vi "Color-Senser-Dtermine-Pro_Api.vi"(8 "Error In":errorcluster, 11 "HiTechnicColorSensorV2 Ref In":cluster{"I2C Ref Out":T2}) -> (0 "Error Out":errorcluster, 1 "Green or Saturation":i32, 2 "對應顏色":enum16{"黃", "紅", "綠", "藍", "黑", "無"}(ring), 3 "HiTechnicColorSensorV2 Ref Out":cluster{"I2C Ref Out":T2}, 4 "Red or Hue":i32, 5 "當前顏色值":T1(array[cluster]))   [LabVIEW 2019]
uses:
  Variable/Indentify-Consequent.vi
  <vilib>/myRIO/Common/Instrument Driver Framework/myRIO v1.0/DIO/typedefs/DIO Channels Enum.ctl
  <vilib>/myRIO/Common/Instrument Driver Framework/myRIO v1.0/DIO/typedefs/DIO Channels List.ctl
  <vilib>/myRIO/Common/Instrument Driver Framework/Utilities/typedefs/Generic FPGA Reference.ctl
  <vilib>/myRIO/Common/Instrument Driver Framework/Utilities/typedefs/myRIO v1.0 Reference.ctl
  <vilib>/myRIO/Common/Instrument Driver Framework/Utilities/typedefs/Hardware Version Enum.ctl
  <vilib>/myRIO/Common/Instrument Driver Framework/Utilities/typedefs/myRIO Generic Hardware Reference.ctl
  <vilib>/myRIO/Instrument Drivers/Onboard IO/DIO/typedefs/DIO Reference.ctl
  <vilib>/myRIO/Instrument Drivers/Onboard IO/DIO/DIO.lvlib
  <vilib>/myRIO/Instrument Drivers/Onboard IO/DIO/vis/Write.vi
  <vilib>/userDefined/High Color/nirio_resource_hc.ctl
  <vilib>/myRIO/Common/Instrument Driver Framework/myRIO v1.0/DIO/vis/myRIO v1.1 Open DIO.vi
  <vilib>/myRIO/Instrument Drivers/Onboard IO/DIO/vis/myRIO DIO Open.xnode
  <vilib>/myRIO/Common/Instrument Driver Framework/Utilities/vis/Is FPGA Ref Available.vi
  <vilib>/myRIO/Express VI/Onboard Devices/LED/LED Express VI.xnode
  <vilib>/myRIO/Common/Instrument Driver Framework/myRIO v1.0/I2C/typedefs/I2C Channels Enum.ctl
  <vilib>/myRIO/Instrument Drivers/Onboard IO/I2C/typedefs/I2C Transfer Rate.ctl
  <vilib>/myRIO/Instrument Drivers/Onboard IO/I2C/I2C.lvlib
  <vilib>/myRIO/Instrument Drivers/Onboard IO/I2C/typedefs/I2C Configuration.ctl
  <vilib>/myRIO/Instrument Drivers/Onboard IO/I2C/typedefs/I2C Reference.ctl
panel:
  in  "Stop":bool
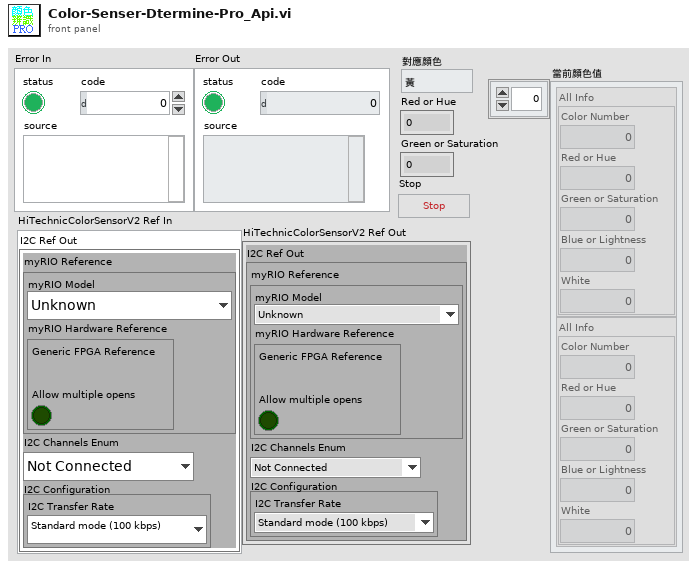
[diagram p1: front panel]
types:
  T1 = cluster{"All Info":cluster{"Color Number":i32, "Red or Hue":i32, "Green or Saturation":i32, "Blue or Lightness":i32, "White":i32}}[]
  T2 = typedef "I2C.lvlib/I2C Reference.ctl" = cluster{"myRIO Reference":T3, "I2C Channels Enum":T7, "I2C Configuration":T8}
  T3 = typedef "myRIO Generic Hardware Reference.ctl" = cluster{"myRIO Model":T4, "myRIO Hardware Reference":T5}
  T4 = typedef "Hardware Version Enum.ctl" = enum16{"Unknown", "myRIO-1900", "myRIO-1950", "roboRIO", "NI ELVIS RIO CM", "ELVIS III"}
  T5 = typedef "myRIO v1.0 Reference.ctl" = cluster{"Generic FPGA Reference":T6, "Allow multiple opens":bool}
  T6 = typedef "Generic FPGA Reference.ctl" = refnum<k20>
  T7 = typedef "I2C Channels Enum.ctl" = enum16{"Not Connected", "A/I2C", "B/I2C", "I2C/I2C"}
  T8 = typedef "I2C.lvlib/I2C Configuration.ctl" = cluster{"I2C Transfer Rate":T9}
  T9 = typedef "I2C.lvlib/I2C Transfer Rate.ctl" = enum16{"Standard mode (100 kbps)", "Fast mode (400 kbps)"}
  T10 = cluster{"All Info":cluster{"Color Number":i32, "Red or Hue":i32, "Green or Saturation":i32, "Blue or Lightness":i32, "White":i32}}
  T11 = typedef "DIO.lvlib/DIO Reference.ctl" = cluster{"myRIO Reference":T3, "DIO Channels List":T12}
  T12 = typedef "DIO Channels List.ctl" = T13[]
  T13 = typedef "DIO Channels Enum.ctl" = enum16{"Not Connected", "C/DIO0", "C/DIO1", "C/DIO2", "C/DIO3", "C/DIO4", "C/DIO5", "C/DIO6", "C/DIO7", "A/DIO0", "A/DIO1", "A/DIO2", "A/DIO3", "A/DIO4", "A/DIO5", "A/DIO6", "A/DIO7", "A/DIO8", "A/DIO9", "A/DIO10", "A/DIO11", "A/DIO12", "A/DIO13", "A/DIO14", "A/DIO15", "A/DIO16", "A/DIO17", "A/DIO18", "A/DIO19", "B/DIO0", "B/DIO1", "B/DIO2", "B/DIO3", "B/DIO4", "B/DIO5", "B/DIO6", "B/DIO7", "B/DIO8", "B/DIO9", "B/DIO10", "B/DIO11", "B/DIO12", "B/DIO13", "B/DIO14", "B/DIO15", "B/DIO16", "B/DIO17", "B/DIO18", "B/DIO19", "LED0", "LED1", "LED2", "LED3", "Button0", "DIO/DIO0", "DIO/DIO1", "DIO/DIO2", "DIO/DIO3", "DIO/DIO4", "DIO/DIO5", "DIO/DIO6", "DIO/DIO7", "DIO/DIO8", "DIO/DIO9", "SPI/CS0", "SPI/CS1", "SPI/CS2", "SPI/CS3", "LED RADIO (Green)", "LED RADIO (Red)", "LED COMM (Green)", "LED COMM (Red)", "LED MODE (Green)", "LED MODE (Red)"}
  T14 = typedef "nirio_resource_hc.ctl" = tag
  T15 = cluster{"Color Number":i32, "Red or Hue":i32, "Green or Saturation":i32, "Blue or Lightness":i32, "White":i32}
  T16 = cluster{"Color Number":dbl, "Red or Hue":dbl, "Green or Saturation":dbl, "Blue or Lightness":dbl, "White":dbl}
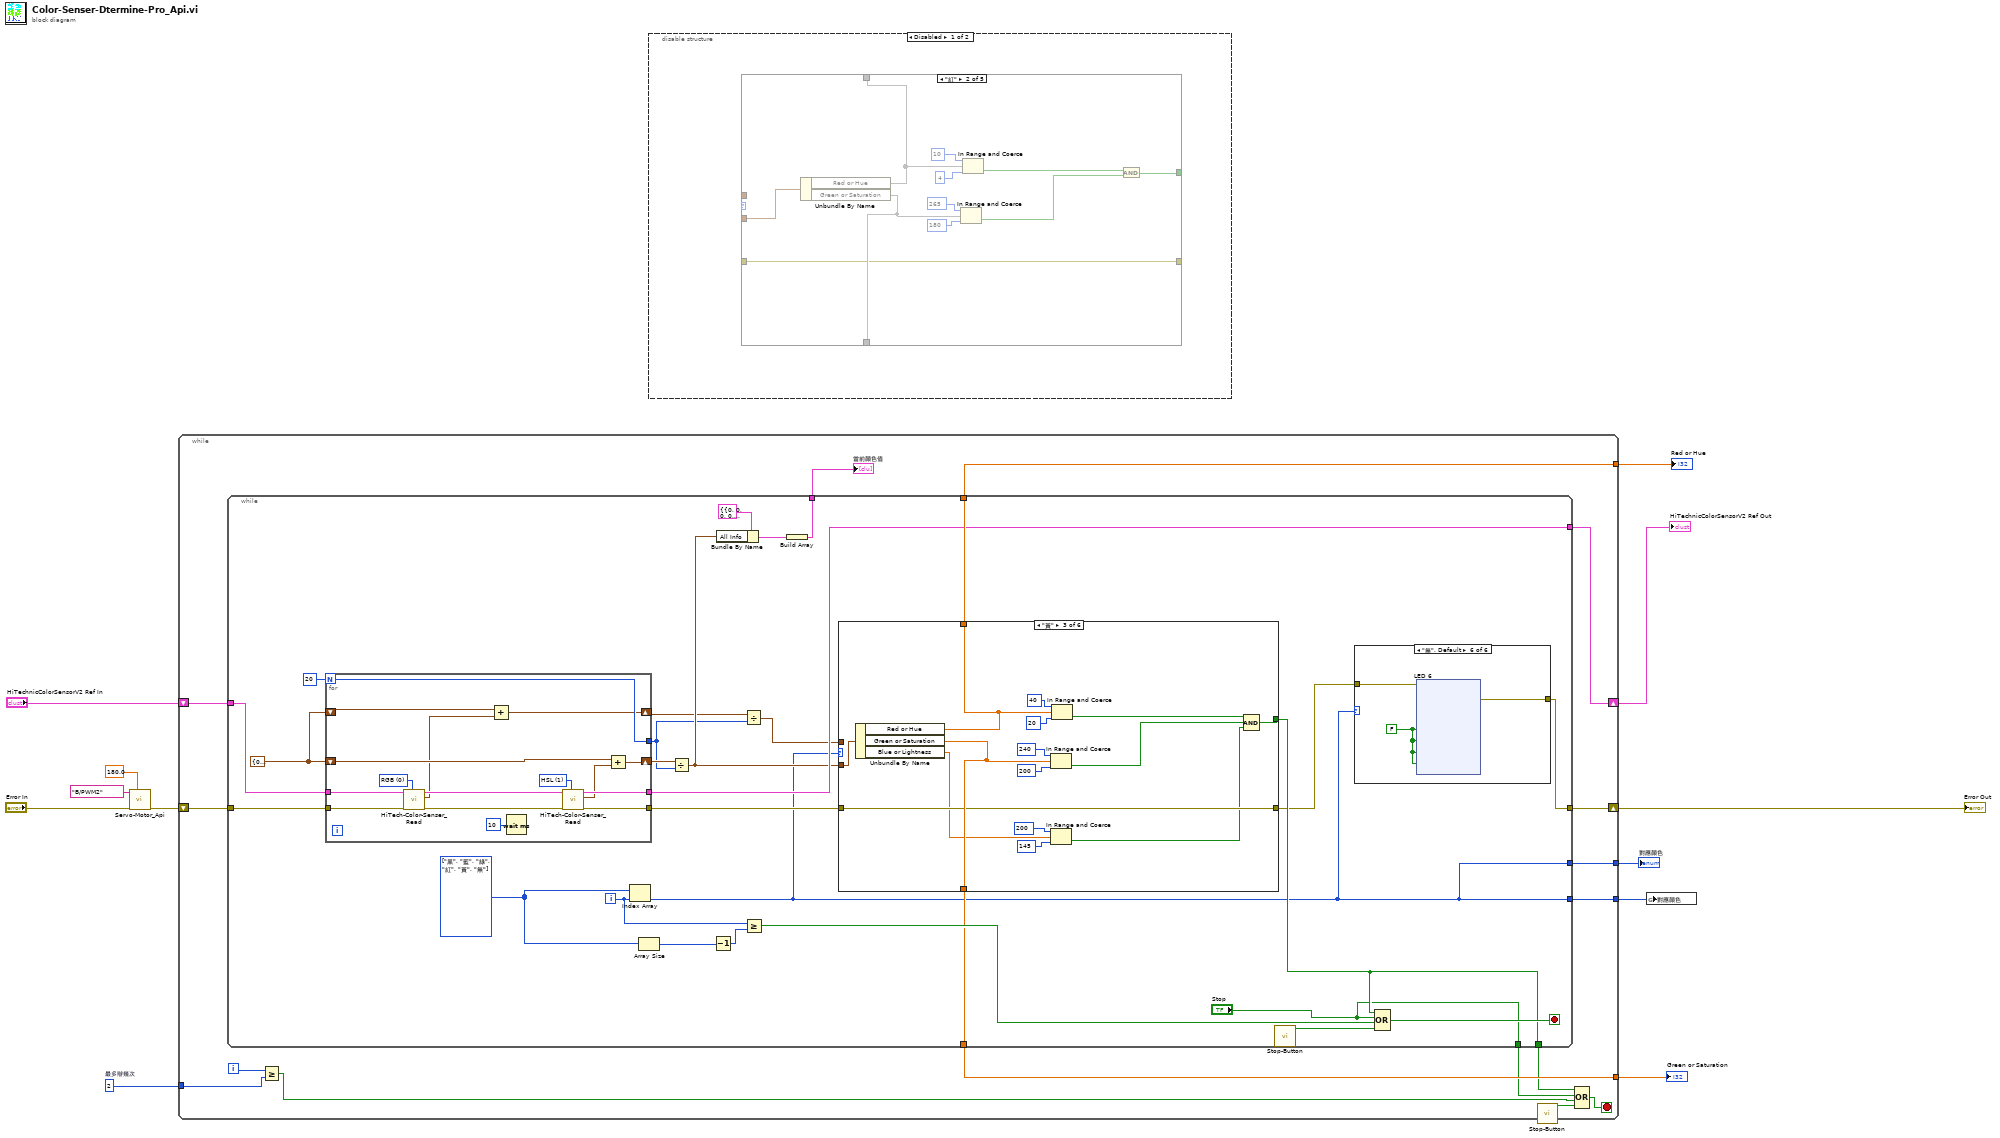
[diagram p0: block diagram]
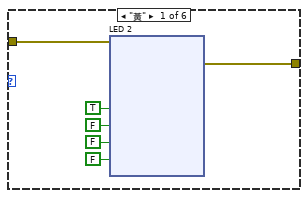
[diagram p2: hidden frame]
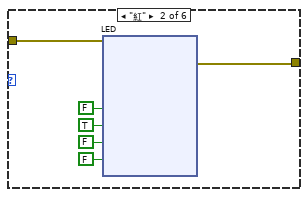
[diagram p3: hidden frame]
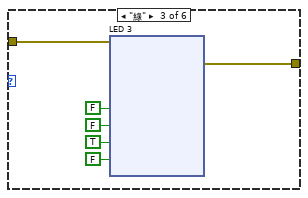
[diagram p4: hidden frame]
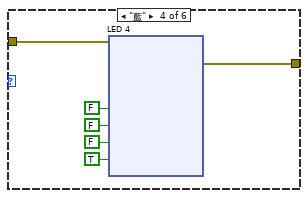
[diagram p5: hidden frame]
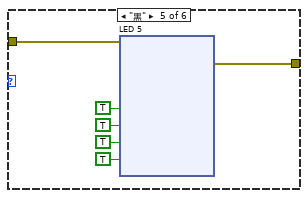
[diagram p6: hidden frame]
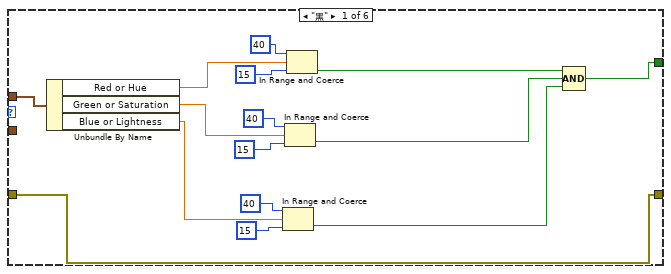
[diagram p7: hidden frame]
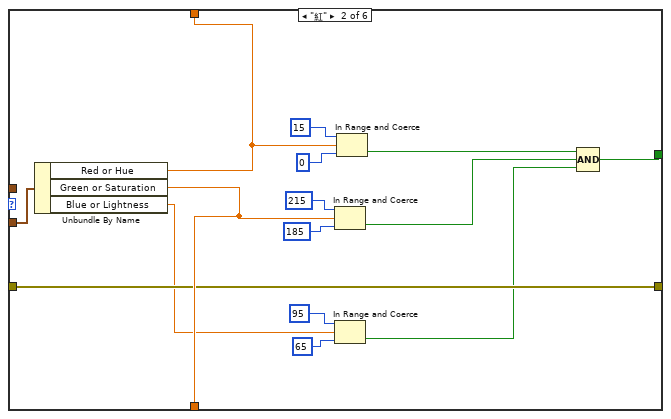
[diagram p8: hidden frame]
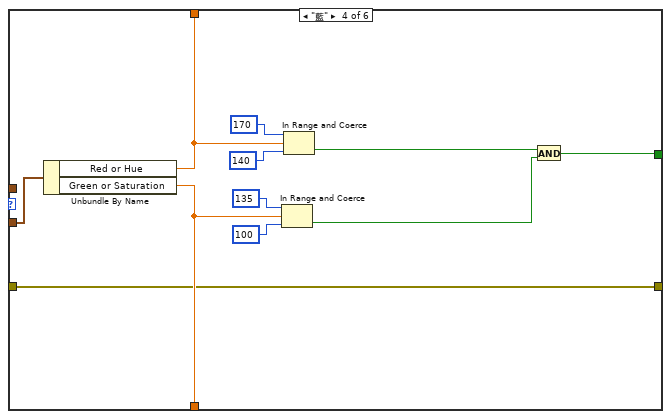
[diagram p9: hidden frame]
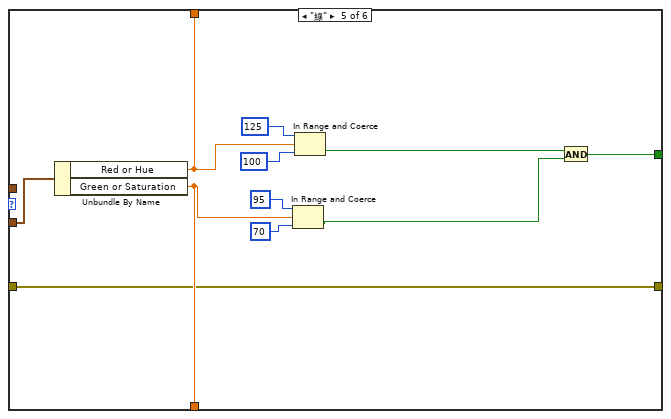
[diagram p10: hidden frame]
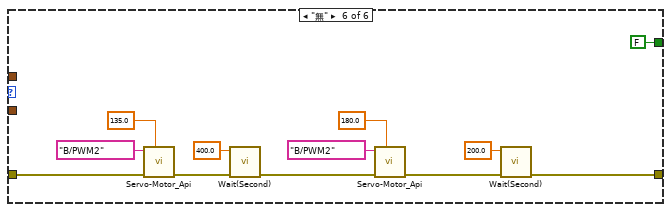
[diagram p11: hidden frame]
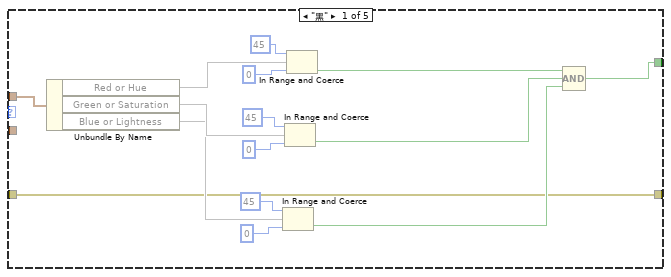
[diagram p12: hidden frame]
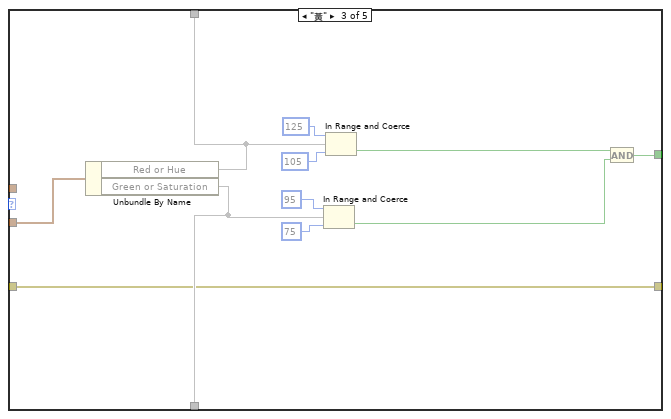
[diagram p13: hidden frame]
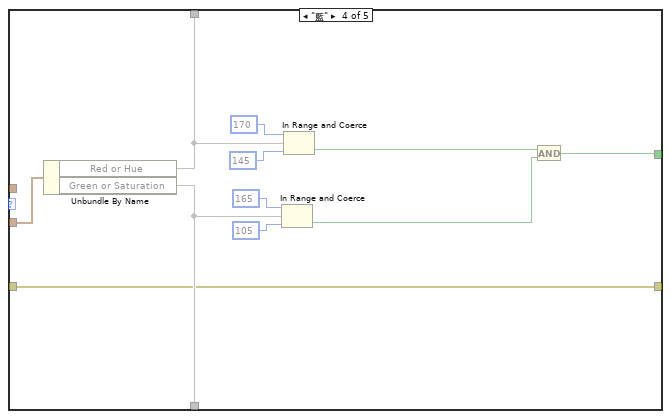
[diagram p14: hidden frame]
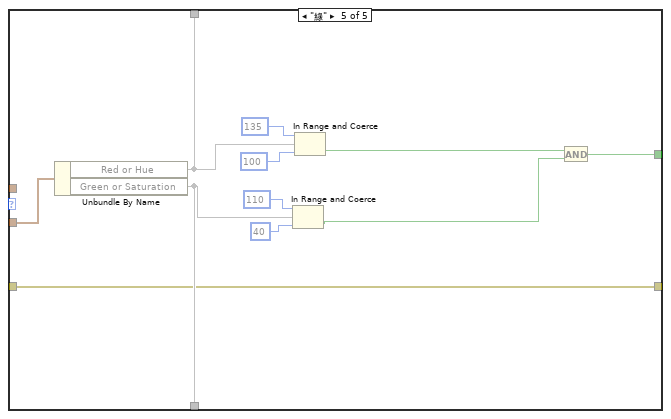
[diagram p15: hidden frame]
diagram:
  w8 = 2  # 最多辯幾次
  n1 = call "Servo-Motor_Api.vi"("角度"=180.0, "Error In"="Error In", "伺服馬達角位"=tag "B/PWM2") -> ("Error Out"=w4:errorcluster)  [unwired: 8 in]
  n2 = while {
    tunnel: [w25] -> w10
    tunnel: [w24] -> w9
    shift-right: [w22] -> w6
    shift-left: w4 -> [w27]
    shift-right: [w28] -> w12
    shift-left: "HiTechnicColorSensorV2 Ref In" -> [w26]
    tunnel: w8 -> [w16]
    tunnel: [w14] -> w7
    tunnel: [w13] -> w5
    i -> [w17]
    stop <- w21 stop-if-true
    n3 = while {
      tunnel: [w31] -> w22
      tunnel: [w44] -> w28
      tunnel: w27 -> [w38]
      tunnel: w26 -> [w39]
      tunnel: [w50] -> w25
      tunnel: [w49] -> w24
      tunnel: [w46] -> w23
      tunnel: [w33] -> w20
      tunnel: ["Stop"] -> w19
      tunnel: [w29] -> w14
      tunnel: [w29] -> w13
      i -> [w45]
      stop <- w53 stop-if-true
      w37 = T15 {"Color Number"=0, "Red or Hue"=0, "Green or Saturation"=0, "Blue or Lightness"=0, "White"=0}
      w54 = enum16{"黃", "紅", "綠", "藍", "黑", "無"}[] [enum."黑", enum."藍", enum."綠", enum."紅", enum."黃", enum."無"] items=["黃", "紅", "綠", "藍", "黑", "無"]
      n4 = for {
        N: 20 -> [w326]
        tunnel: w38 -> [w324]
        tunnel: w39 -> [w325]
        tunnel: [w332] -> w42
        tunnel: [w331] -> w44
        shift-right: [w329] -> w43
        shift-left: w37 -> [w328]
        tunnel: [w326] -> w35
        shift-right: [w319] -> w36
        shift-left: w37 -> [w318]
        w321 = u16 0 items=["RGB", "HSL", "HSV", "HSI", "CIE L*a*b*", "CIE XYZ"] ("Color Mode")
        w333 = u16 1 items=["RGB", "HSL", "HSV", "HSI", "CIE L*a*b*", "CIE XYZ"] ("Color Mode")
        n5 = call "HiTech-Color-Senser_Read.vi"("Color Mode"=w321, "Error In"=w324, "HiTechnicColorSensorV2 Ref In"=w325) -> ("Error Out"=w322:errorcluster, "All Info"=w320:T15, "HiTechnicColorSensorV2 Ref Out"=w323:cluster{"I2C Ref Out":T2})  [unwired: 6 in]
        n6 = Add(x=w318, y=w320) -> (x+y=w319:T15)
        n7 = Wait (ms)(milliseconds to wait=u32 10) -> ()  [unwired: 1 out]
        n8 = call "HiTech-Color-Senser_Read.vi"("Color Mode"=w333, "Error In"=w322, "HiTechnicColorSensorV2 Ref In"=w323) -> ("Error Out"=w332:errorcluster, "All Info"=w330:T15, "HiTechnicColorSensorV2 Ref Out"=w331:cluster{"I2C Ref Out":T2})  [unwired: 6 in]
        n9 = Add(x=w328, y=w330) -> (x+y=w329:T15)
      }
      n10 = Index Array(array=w54, index=w45) -> (element=w29:enum16{"黃", "紅", "綠", "藍", "黑", "無"})
      n11 = Array Size(array=w54) -> (size(s)=w56:i32)
      n12 = Divide(x=w43, y=w35) -> (x/y=w41:T16)
      n13 = Decrement(x=w56) -> (x-1=w55:i32)
      n14 = Bundle By Name(cluster=T10 {"All Info"={"Color Number"=0, "Red or Hue"=0, "Green or Saturation"=0, "Blue or Lightness"=0, "White"=0}} ("input cluster"), "All Info"=w41) -> (w48:T10)
      n15 = Divide(x=w36, y=w35) -> (x/y=w34:T16)
      n16 = Greater Or Equal?(x=w45, y=w55) -> (x >= y?=w52:bool)
      n17 = Build Array(w48) -> (w46:T1)
      n18 = case shown="\"黃\"" w29 {
        tunnel: w34 -> [w342 _ _ _ _ _]
        tunnel: [w334 w357 w372 w383 w394 FALSE] -> w33
        tunnel: [_ w356 w371 w381 w393 _] -> w50
        tunnel: [_ w355 w370 w382 w392 _] -> w49
        tunnel: [w335 w354 w369 w380 w391 w401] -> w30
        tunnel: w42 -> [w335 w354 w369 w380 w391 w411]
        tunnel: w41 -> [_ w353 w368 w379 w390 _]
        frame "黑" {
          n19 = Unbundle By Name(w342) -> ("Red or Hue"=w348:dbl, "Green or Saturation"=w347:dbl, "Blue or Lightness"=w339:dbl)
          n20 = In Range and Coerce(upper limit=40, x=w339, lower limit=15) -> (In Range?=w336:bool)  [unwired: 1 out]
          n21 = In Range and Coerce(upper limit=40, x=w347, lower limit=15) -> (In Range?=w337:bool)  [unwired: 1 out]
          n22 = In Range and Coerce(upper limit=40, x=w348, lower limit=15) -> (In Range?=w338:bool)  [unwired: 1 out]
          n23 = Compound Arithmetic op=AND(w338, w337, w336) -> (w334:bool)
        }
        frame "紅" {
          n24 = Unbundle By Name(w353) -> ("Red or Hue"=w356:dbl, "Green or Saturation"=w355:dbl, "Blue or Lightness"=w349:dbl)
          n25 = In Range and Coerce(upper limit=215, x=w355, lower limit=185) -> (In Range?=w358:bool)  [unwired: 1 out]
          n26 = In Range and Coerce(upper limit=95, x=w349, lower limit=65) -> (In Range?=w350:bool)  [unwired: 1 out]
          n27 = In Range and Coerce(upper limit=15, x=w356, lower limit=0) -> (In Range?=w359:bool)  [unwired: 1 out]
          n28 = Compound Arithmetic op=AND(w359, w358, w350) -> (w357:bool)
        }
        frame "黃" {
          n29 = Unbundle By Name(w368) -> ("Red or Hue"=w371:dbl, "Green or Saturation"=w370:dbl, "Blue or Lightness"=w364:dbl)
          n30 = In Range and Coerce(upper limit=240, x=w370, lower limit=200) -> (In Range?=w373:bool)  [unwired: 1 out]
          n31 = In Range and Coerce(upper limit=200, x=w364, lower limit=145) -> (In Range?=w365:bool)  [unwired: 1 out]
          n32 = In Range and Coerce(upper limit=40, x=w371, lower limit=20) -> (In Range?=w374:bool)  [unwired: 1 out]
          n33 = Compound Arithmetic op=AND(w374, w373, w365) -> (w372:bool)
        }
        frame "藍" {
          n34 = Unbundle By Name(w379) -> ("Red or Hue"=w381:dbl, "Green or Saturation"=w382:dbl)
          n35 = In Range and Coerce(upper limit=135, x=w382, lower limit=100) -> (In Range?=w384:bool)  [unwired: 1 out]
          n36 = In Range and Coerce(upper limit=170, x=w381, lower limit=140) -> (In Range?=w385:bool)  [unwired: 1 out]
          n37 = And(x=w385, y=w384) -> (x .and. y?=w383:bool)
        }
        frame "綠" {
          n38 = Unbundle By Name(w390) -> ("Red or Hue"=w393:dbl, "Green or Saturation"=w392:dbl)
          n39 = In Range and Coerce(upper limit=95, x=w392, lower limit=70) -> (In Range?=w395:bool)  [unwired: 1 out]
          n40 = In Range and Coerce(upper limit=125, x=w393, lower limit=100) -> (In Range?=w396:bool)  [unwired: 1 out]
          n41 = And(x=w396, y=w395) -> (x .and. y?=w394:bool)
        }
        frame "無" {
          n42 = call "Servo-Motor_Api.vi"("角度"=135.0, "Error In"=w411, "伺服馬達角位"=tag "B/PWM2") -> ("Error Out"=w410:errorcluster)  [unwired: 8 in]
          n43 = call "Wait(Second).vi"("Error In"=w410, "等待秒數(3000毫秒)"=400.0) -> ("Error Out"=w404:errorcluster)  [unwired: 9 in]
          n44 = call "Servo-Motor_Api.vi"("角度"=180.0, "Error In"=w404, "伺服馬達角位"=tag "B/PWM2") -> ("Error Out"=w402:errorcluster)  [unwired: 8 in]
          n45 = call "Wait(Second).vi"("Error In"=w402, "等待秒數(3000毫秒)"=200.0) -> ("Error Out"=w401:errorcluster)  [unwired: 9 in]
        }
      }
      n46 = call "Stop-Button.vi"() -> ("顯示按下?"=w51:bool)  [unwired: 10 in, 1 out]
      n47 = case shown="\"無\", Default" w29 {
        tunnel: w30 -> [w58 w102 w146 w190 w234 w279]
        tunnel: [w57 w101 w145 w189 w233 w278] -> w31
        frame "黃" {
          n48 = xnode "LED 2"("LED0"=TRUE, "LED1"=FALSE, "LED2"=FALSE, "LED3"=FALSE, "error in (no error)"=w58) -> ("error out"=w57:errorcluster)
        }
        frame "紅" {
          n49 = xnode "LED"("LED0"=FALSE, "LED1"=TRUE, "LED2"=FALSE, "LED3"=FALSE, "error in (no error)"=w102) -> ("error out"=w101:errorcluster)
        }
        frame "綠" {
          n50 = xnode "LED 3"("LED0"=FALSE, "LED1"=FALSE, "LED2"=TRUE, "LED3"=FALSE, "error in (no error)"=w146) -> ("error out"=w145:errorcluster)
        }
        frame "藍" {
          n51 = xnode "LED 4"("LED0"=FALSE, "LED1"=FALSE, "LED2"=FALSE, "LED3"=TRUE, "error in (no error)"=w190) -> ("error out"=w189:errorcluster)
        }
        frame "黑" {
          n52 = xnode "LED 5"("LED0"=TRUE, "LED1"=TRUE, "LED2"=TRUE, "LED3"=TRUE, "error in (no error)"=w234) -> ("error out"=w233:errorcluster)
        }
        frame "無", Default {
          w277 = FALSE ("LED0")
          n53 = xnode "LED 6"("LED0"=w277, "LED1"=w277, "LED2"=w277, "LED3"=w277, "error in (no error)"=w279) -> ("error out"=w278:errorcluster)
        }
      }
      n54 = Compound Arithmetic op=OR(w33, "Stop", w52, w51) -> (w53:bool)
    }
    "當前顏色值" <- w23
    n55 = Greater Or Equal?(x=w17, y=w16) -> (x >= y?=w15:bool)
    n56 = call "Stop-Button.vi"() -> ("顯示按下?"=w18:bool)  [unwired: 10 in, 1 out]
    n57 = Compound Arithmetic op=OR(w20, w19, w15, w18) -> (w21:bool)
  }
  "Error Out" <- w6
  "HiTechnicColorSensorV2 Ref Out" <- w12
  "Red or Hue" <- w10
  "Green or Saturation" <- w9
  "對應顏色" <- w5
  n58 = disable-structure shown="Disabled" {
    frame Disabled {
      n59 = case shown="\"紅\"" {
        selector: _ -> [_ _ _ _ _]
        tunnel: _ -> [w421 _ _ _ _]
        tunnel: [w413 w432 w443 w454 w465] -> _
        tunnel: [_ w431 w442 w452 w464] -> _
        tunnel: [_ w430 w441 w453 w463] -> _
        tunnel: [w414 w429 w440 w451 w462] -> _
        tunnel: _ -> [w414 w429 w440 w451 w462]
        tunnel: _ -> [_ w428 w439 w450 w461]
        frame "黑" {
          n60 = Unbundle By Name(w421) -> ("Red or Hue"=w427, "Green or Saturation"=w426, "Blue or Lightness"=w418)
          n61 = In Range and Coerce(upper limit=45, x=w418, lower limit=0) -> (In Range?=w415:bool)  [unwired: 1 out]
          n62 = In Range and Coerce(upper limit=45, x=w426, lower limit=0) -> (In Range?=w416:bool)  [unwired: 1 out]
          n63 = In Range and Coerce(upper limit=45, x=w427, lower limit=0) -> (In Range?=w417:bool)  [unwired: 1 out]
          n64 = Compound Arithmetic op=AND(w417, w416, w415) -> (w413:bool)
        }
        frame "紅" {
          n65 = Unbundle By Name(w428) -> ("Red or Hue"=w431, "Green or Saturation"=w430)
          n66 = In Range and Coerce(upper limit=265, x=w430, lower limit=180) -> (In Range?=w433:bool)  [unwired: 1 out]
          n67 = In Range and Coerce(upper limit=10, x=w431, lower limit=4) -> (In Range?=w434:bool)  [unwired: 1 out]
          n68 = And(x=w434, y=w433) -> (x .and. y?=w432:bool)
        }
        frame "黃" {
          n69 = Unbundle By Name(w439) -> ("Red or Hue"=w442, "Green or Saturation"=w441)
          n70 = In Range and Coerce(upper limit=95, x=w441, lower limit=75) -> (In Range?=w444:bool)  [unwired: 1 out]
          n71 = In Range and Coerce(upper limit=125, x=w442, lower limit=105) -> (In Range?=w445:bool)  [unwired: 1 out]
          n72 = And(x=w445, y=w444) -> (x .and. y?=w443:bool)
        }
        frame "藍" {
          n73 = Unbundle By Name(w450) -> ("Red or Hue"=w452, "Green or Saturation"=w453)
          n74 = In Range and Coerce(upper limit=165, x=w453, lower limit=105) -> (In Range?=w455:bool)  [unwired: 1 out]
          n75 = In Range and Coerce(upper limit=170, x=w452, lower limit=145) -> (In Range?=w456:bool)  [unwired: 1 out]
          n76 = And(x=w456, y=w455) -> (x .and. y?=w454:bool)
        }
        frame "綠" {
          n77 = Unbundle By Name(w461) -> ("Red or Hue"=w464, "Green or Saturation"=w463)
          n78 = In Range and Coerce(upper limit=110, x=w463, lower limit=40) -> (In Range?=w466:bool)  [unwired: 1 out]
          n79 = In Range and Coerce(upper limit=135, x=w464, lower limit=100) -> (In Range?=w467:bool)  [unwired: 1 out]
          n80 = And(x=w467, y=w466) -> (x .and. y?=w465:bool)
        }
      }
    }
    frame Enabled {
    }
  }
  n81 = global write "Indentify-Consequent.vi" "對應顏色"(w7) -> ()
